vi "DynamicRange.vi"(10 "MaxIndex":i32, 11 "Power (dBm)":dbl[](array[numeric])) -> (1 "median":dbl format="%0.2f", 2 "DynamicRange":dbl)   [LabVIEW 2018]
uses:
  <vilib>/Analysis/NI_AALBase.lvlib
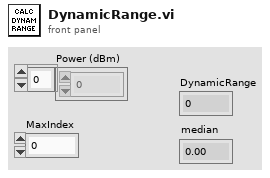
[diagram p1: front panel]
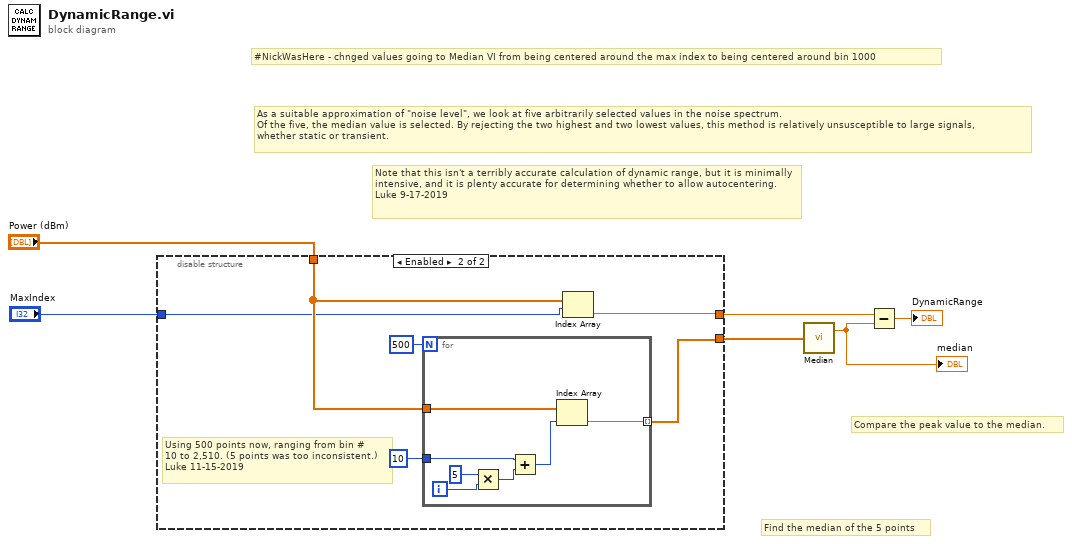
[diagram p0: block diagram]
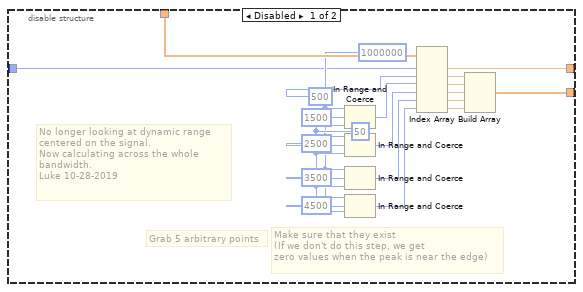
[diagram p2: hidden frame]
diagram:
  # "#NickWasHere - chnged values going to Median VI from being centered around the max index to being centered around bin 1000"
  # "Note that this isn't a terribly accurate calculation of dynamic range, but it is minimally intensive, and it is plenty accurate for determining whether to allow autocentering. Luke 9-17-2019"
  # "Compare the peak value to the median."
  # "Find the median of the 5 points"
  # "As a suitable approximation of \"noise level\", we look at five arbitrarily selected values in the noise spectrum.\nOf the five, the median value is selected. By rejecting the two highest and two lowest values, this method is relatively unsusceptible to large signals,\nwhether static or transient."
  n1 = disable-structure shown="Enabled" {
    disable-tunnel: "Power (dBm)" -> [w26 w31]
    disable-tunnel: [w15 w27] -> w5
    disable-tunnel: [w14 w28] -> w4
    disable-tunnel: "MaxIndex" -> [w7 w30]
    frame Disabled {
      w8 = 1000000 ("upper limit")
      w9 = 50 ("lower limit")
      # "No longer looking at dynamic range\ncentered on the signal.\nNow calculating across the whole\nbandwidth.\nLuke 10-28-2019"
      # "Make sure that they exist\n(If we don't do this step, we get\nzero values when the peak is near the edge)"
      # "Grab 5 arbitrary points"
      n2 = In Range and Coerce(upper limit=w8, x=1500, lower limit=w9) -> (coerced(x)=w10:i32)  [unwired: 1 out]
      n3 = In Range and Coerce(upper limit=w8, x=2500, lower limit=w9) -> (coerced(x)=w11:i32)  [unwired: 1 out]
      n4 = In Range and Coerce(upper limit=w8, x=3500, lower limit=w9) -> (coerced(x)=w12:i32)  [unwired: 1 out]
      n5 = In Range and Coerce(upper limit=w8, x=4500, lower limit=w9) -> (coerced(x)=w13:i32)  [unwired: 1 out]
      n6 = Index Array(array=w26, index #1=w7, index #2=500, index #3=w10, index #4=w11, index #5=w12, index #6=w13) -> (element #1=w14:dbl, element #2=w20:dbl, element #3=w19:dbl, element #4=w18:dbl, element #5=w17:dbl, element #6=w16:dbl)
      n7 = Build Array(w20, w19, w18, w17, w16) -> (w15:dbl[])
    }
    frame Enabled {
      # "Using 500 points now, ranging from bin #\n10 to 2,510. (5 points was too inconsistent.)\nLuke 11-15-2019"
      n8 = for {
        N: 500 -> [_]
        tunnel: w31 -> [w39]
        tunnel: 10 ("x") -> [w35]
        tunnel: [w33] -> w27 mode=indexing
        i -> [w38]
        n9 = Multiply(x=5, y=w38) -> (x*y=w36:i32)
        n10 = Add(x=w35, y=w36) -> (x+y=w34:i32)
        n11 = Index Array(array=w39, index=w34) -> (element=w33:dbl)
      }
      n12 = Index Array(array=w31, index=w30) -> (element=w28:dbl)
    }
  }
  n13 = call <vilib>:"Median.vi"("X"=w5) -> ("median"=w3:dbl)  [unwired: 1 out]
  "median" <- w3
  n14 = Subtract(x=w4, y=w3) -> (x-y=→"DynamicRange":dbl)
